vi "Get All SetList Display Info.vi"(0 "Devices":refnum<class "Device.lvclass">[](array[class])) -> (1 "Columns":refnum<class "Column.lvclass">[](array[class]), 2 "DevNums":i32[](array[numeric]), 3 "Table Data":string[][](array[string]))   [LabVIEW 2013]
uses:
  Device/Device.lvclass
  ColumnVIs/Column/Column.lvclass
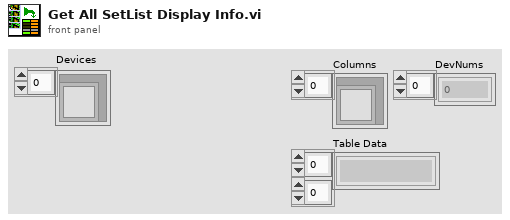
[diagram p1: front panel]
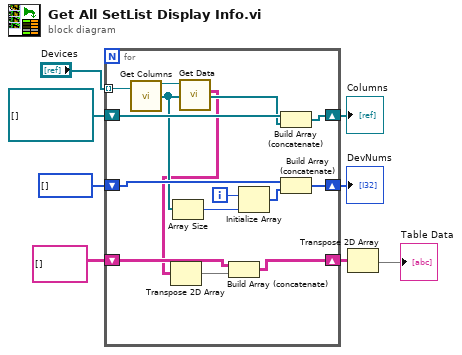
[diagram p0: block diagram]
diagram:
  n1 = for {
    tunnel: "Devices" -> [w22] mode=indexing
    shift-right: [w20] -> w5
    shift-left: refnum<class "Column.lvclass">[] [] ("Columns") -> [w21]
    shift-right: [w15] -> w4
    shift-left: i32[] [] -> [w16]
    shift-right: [w9] -> w2
    shift-left: string[][] [] ("Table Control") -> [w12]
    i -> [w18]
    n2 = call-dynamic "Get Columns.vi"("Device in"=w22) -> ("Device out"=w13:refnum<class "Device.lvclass">, "Columns"=w14:refnum<class "Column.lvclass">[])  [unwired: 1 in, 1 out]
    n3 = Array Size(array=w14) -> (size(s)=w19:i32)
    n4 = call-dynamic "Get Data.vi"("Device in"=w13) -> ("Table Indicator"=w11:string[][])  [unwired: 7 in, 2 out]
    n5 = Transpose 2D Array(2D array=w11) -> (transposed array=w10:string[][])
    n6 = Build Array (concatenate)(w12, w10) -> (w9:string[][])
    n7 = Initialize Array(w18, w19) -> (w17:i32[])
    n8 = Build Array (concatenate)(w21, w14) -> (w20:refnum<class "Column.lvclass">[])
    n9 = Build Array (concatenate)(w16, w17) -> (w15:i32[])
  }
  "Columns" <- w5
  "DevNums" <- w4
  n10 = Transpose 2D Array(2D array=w2) -> (transposed array=→"Table Data":string[][])
